vi "Remove Batch Nodes.vi"(8 "error in (no error)":errorcluster, 9 "Actors ID":variant[](array[variant]), 10 "Timeout(ms)":i64=1000, 11 "Simple Numeric Map Node Controller in":refnum<class "Simple Numeric Map Node Controller.lvclass">) -> (0 "error out":errorcluster, 3 "Simple Numeric Map Node Controller out":refnum<class "Simple Numeric Map Node Controller.lvclass">)   [LabVIEW 2024, in "Simple Numeric Map Node Controller.lvclass"]
uses:
  Simple Numeric Map Node Controller.lvclass
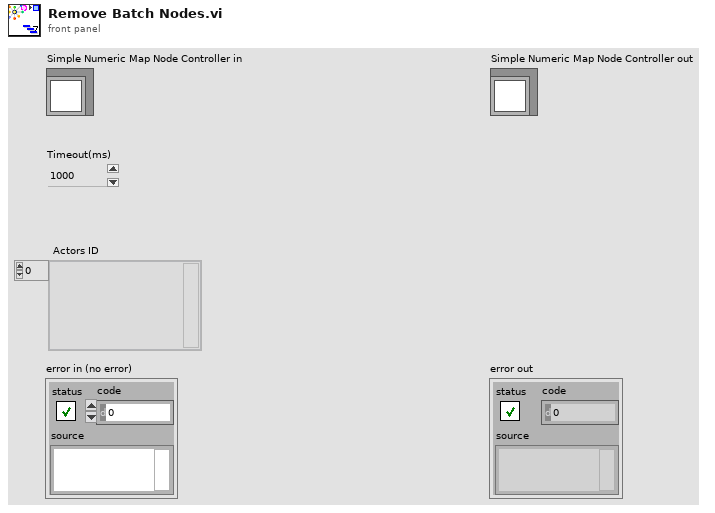
[diagram p1: front panel]
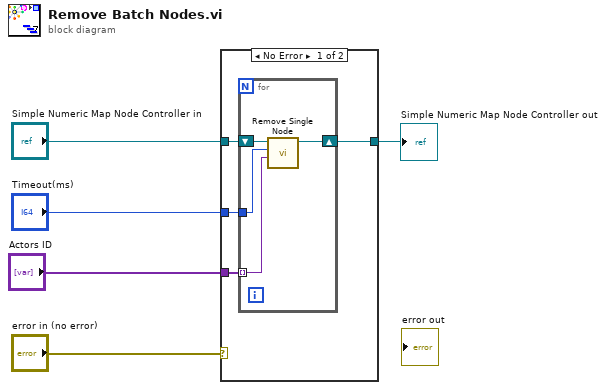
[diagram p0: block diagram]
diagram:
  n1 = case shown="No Error" "error in (no error)" {
    tunnel: "Simple Numeric Map Node Controller in" -> [w9 w14]
    tunnel: [w8 w14] -> w4
    tunnel: "Timeout(ms)" -> [w7 _]
    tunnel: "Actors ID" -> [w6 _]
    frame No Error {
      n2 = for {
        shift-right: [w12] -> w8
        shift-left: w9 -> [w13]
        tunnel: w7 -> [w11]
        tunnel: w6 -> [w10] mode=indexing
        n3 = call-dynamic "Remove Single Node.vi"("Actor ID"=w10, "Timeout(ms)"=w11, "Simple Numeric Map Node Controller in"=w13) -> ("Simple Numeric Map Node Controller out"=w12:refnum<class "Simple Numeric Map Node Controller.lvclass">)  [unwired: 7 in, 1 out]
      }
    }
    frame Error {
    }
  }
  "Simple Numeric Map Node Controller out" <- w4
